vi "Default Instrument Setup.vi"(8 "error in (no error)":errorcluster, 11 "VISA resource name":refnum<visa-resource-name>) -> (0 "error out":errorcluster, 3 "VISA resource name out":refnum<visa-resource-name>)   [LabVIEW 2012, in "Agilent 8000 Series.lvlib"]
doc: "This Utility VI sends a default command string to the instrument whenever a new VISA session is opened, or the instrument is reset. Use this VI as a subVI for the Initialize and Reset VIs. Altering this VI could cause these two VIs to operate incorrectly."
uses:
  <instrlib>/Agilent 8000 Series/Agilent 8000 Series.lvlib
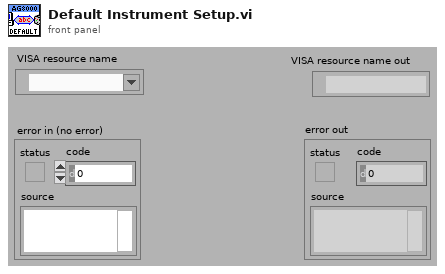
[diagram p1: front panel]
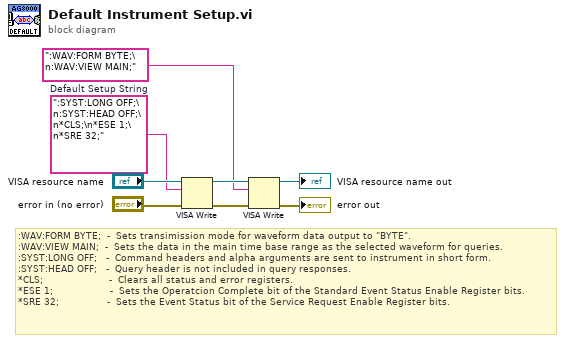
[diagram p0: block diagram]
diagram:
  w6 = ":SYST:LONG OFF;\n:SYST:HEAD OFF;\n*CLS;\n*ESE 1;\n*SRE 32;"  # Default Setup String
  # ":WAV:FORM BYTE;  -  Sets transimission mode for waveform data output to \"BYTE\".\n:WAV:VIEW MAIN;  -  Sets the data in the main time base range as the selected waveform for queries.\n:SYST:LONG OFF;   -  Command headers and alpha arguments are sent to instrument in short form.\n:SYST:HEAD OFF;   -  Query header is not included in query responses.\n*CLS;                      -  Clears all status and error registers.\n*ESE 1;                   -  Sets the Operatcion Complete bit of the Standard Event Status Enable Register bits.\n*SRE 32;                -  Sets the Event Status bit of the Service Request Enable Register bits."
  n1 = VISA Write(VISA resource name="VISA resource name", write buffer=w6, error in (no error)="error in (no error)") -> (VISA resource name out=w5:refnum<visa-resource-name>, error out=w4:errorcluster)  [unwired: 1 out]
  n2 = VISA Write(VISA resource name=w5, write buffer=":WAV:FORM BYTE;\n:WAV:VIEW MAIN;", error in (no error)=w4) -> (VISA resource name out=→"VISA resource name out":refnum<visa-resource-name>, error out=→"error out":errorcluster)  [unwired: 1 out]
